vi "zoss control v1 (top level vi).vi"() -> ()   [LabVIEW 2021]
uses:
  <vilib>/Utility/error.llb/DialogType.ctl
  <vilib>/ErrorRing/Error Ring.xnode
  <vilib>/Utility/error.llb/Error Cluster From Error Code.vi
  global-variables/global variables.vi
  <extravilib>/ChannelInstances/Tag-bool.lvlib
  type-defs/maim stimulation ui states.ctl
  <vilib>/DAQmx/write.llb/DAQmx Write (Digital 1D Bool NChan 1Samp 1Line).vi
  <vilib>/DAQmx/write.llb/DAQmx Write (Digital U32 1Chan 1Samp).vi
  type-defs/stim timestamp cluster (type def).ctl
  <extravilib>/ChannelInstances/Tag-t'stim timestamp cluster (type def).ctl'.lvlib
  <extravilib>/ChannelInstances/Stream-t'sensirion_data_with_time.ctl'.lvlib
  <extravilib>/ChannelInstances/Tag-c(i32,bool).lvlib
  <vilib>/Analysis/NI_AALPro.lvlib
  <vilib>/Analysis/NI_AALBase.lvlib
  type-defs/cam_2p_status_logging_states.ctl
  <vilib>/DAQmx/read.llb/DAQmx Read (Digital 1D Bool NChan 1Samp 1Line).vi
  <vilib>/Analysis/baseanly.llb/Mean (DBL).vi
  type-defs/odor color (type def).ctl
  type-defs/stimulation configuration array (type def).ctl
  type-defs/stimulator configuration line cluster (type def).ctl
  type-defs/port-odor with color cluster (type def).ctl
  type-defs/port-odor ring (type def).ctl
  type-defs/odor and manifold config cluster (type def).ctl
  type-defs/manifold configuration cluster array (type def).ctl
  type-defs/manifold configuration cluster (type def).ctl
  type-defs/manifold selection.ctl
  type-defs/single port single odor cluster.ctl
  type-defs/port number (type def).ctl
  type-defs/odor selection (type def).ctl
  type-defs/odor description array (type def).ctl
  type-defs/odor info cluster (type def).ctl
  controls/sensirion_flow_sensor_data.ctl
  controls/sensirion_flow_sensor_data (small).ctl
panel:
  in  "DAQmx Device Name 7":tag="Dev1-USB6259"
  in  "DAQmx Device Name 6":tag="Dev1-USB6259"
  in  "DAQmx Device Name 5":tag="Dev1-USB6259"
  in  "DAQmx Device Name 4":tag="Dev1-USB6259"
  in  "DAQmx Device Name 3":tag="Dev1-USB6259"
  in  "DAQmx Device Name 2":tag="Dev1-USB6259"
  out "main progress bar":dbl(slide) scale=0.0..1.0
  out "est stim. time, s 2":dbl caption="Estimated Stimulation Duration" format="(%.0f s)"
  out "est stim. time, s":dbl caption="Estimated Stimulation Duration" format="%<%H h, %M m, %S s>t"
  out "Manual Sync":bool
  out "CAM Status":bool
  out "2P Status":bool
  out "stimulation":bool
  out "elapsed stim. time":dbl caption="Elapsed Stimulation Time" format="%<%H h, %M m, %S%1u s>t"
  out "app running":bool
  out "time":timestamp format="%<%H:%M:%S\n%x>T"
  out "experiment directory":path
  out "experiment name":string
  in  "start button":bool
  in  "quit button":bool
  in  "Tab Control":T1(tab)
  out "stim progress bar":dbl(slide)
  in  "trig on btn":bool
  in  "sol. off btn.":bool
  in  "trig off btn":bool
  in  "Trigger Selection":T2={"Trig. 0"=TRUE, "Trig. 1"=FALSE, "Trig. 2"=FALSE, "Trig. 3"=FALSE}
  out "stim duration":dbl caption="Duration" format="%<%M:%S%1u>t"
  out "Triggers":T2
  out "Stimulation Step":string
  in  "DAQmx Device Name":tag="Dev1-USB6259"
  out "Solenoid Status":T3
  out "stim status mc listbox":i32(listbox)=-1 caption="Stimulation Sequence & Status"
  out "stim loop state":T4
  in  "pre-trig pause, s (5)":dbl=5.0 caption="Pre-Trigger Pause" format="%.1f s"
  out "time left (s)":dbl caption="Time Left" format="%<%M:%S%1u>t"
  in  "post-stim pause, s (3)":dbl=3.0 caption="Post-Stimulation Pause" format="%.1f s"
  out "stim log path":path caption="Stimulation Logfile Path"
  in  "stim. run num.":i32=1 caption="Next Stimulation Run Index" format="%03d"
  out "stim. config array":T5 caption="Stimulation Sequence Configuration" {"right odor"."port-odor ring" items=["off"]; "middle odor"."port-odor ring" items=["off"=0, "fish-water (Odor: 2, Port: M.1)"=2]; "left odor"."port-odor ring" items=["off"]}
  in  "config stim button":bool
  out "odor & manifold config cluster":T10
  in  "config odor-manifold button":bool
  in  "dish volume live?":bool=TRUE caption="Live Volume"
  in  "dish volume input":dbl[unit] format="%0.2f"
  out "dish vol.":dbl[unit](slide) caption="Dish Volume (mL)"
  out "sensor uptime":dbl[unit] caption="Sensor Log Up-Time" format="%<%H h, %M m, %S%1u s>t"
  out "Sensor Status":errorcluster
  in  "sensor monitor stop-start":bool
  out "wash-vac delta":dbl[unit](slide) caption="Dish Net Flow Rate"
  out "10 sensor data clustor":T20={"sensor 0"={"flow rate \n"=0.0, "flow val. status"=FALSE, "temperature"=273.15, "temp. val status"=FALSE, "air in line?"=FALSE, "high flow?"=FALSE, "flag. val status"=FALSE}, "sensor 1"={"flow rate \n"=0.0, "flow val. status"=FALSE, "temperature"=273.15, "temp. val status"=FALSE, "air in line?"=FALSE, "high flow?"=FALSE, "flag. val status"=FALSE}, "sensor 2"={"flow rate \n"=0.0, "flow val. status"=FALSE, "temperature"=273.15, "temp. val status"=FALSE, "air in line?"=FALSE, "high flow?"=FALSE, "flag. val status"=FALSE}, "sensor 3"={"flow rate \n"=0.0, "flow val. status"=FALSE, "temperature"=273.15, "temp. val status"=FALSE, "air in line?"=FALSE, "high flow?"=FALSE, "flag. val status"=FALSE}, "sensor 4"={"flow rate \n"=0.0, "flow val. status"=FALSE, "temperature"=273.15, "temp. val status"=FALSE, "air in line?"=FALSE, "high flow?"=FALSE, "flag. val status"=FALSE}, "sensor 5"={"flow rate \n"=0.0, "flow val. status"=FALSE, "temperature"=273.15, "temp. val status"=FALSE, "air in line?"=FALSE, "high flow?"=FALSE, "flag. val status"=FALSE}, "sensor 6"={"flow rate \n"=0.0, "flow val. status"=FALSE, "temperature"=273.15, "temp. val status"=FALSE, "air in line?"=FALSE, "high flow?"=FALSE, "flag. val status"=FALSE}, "sensor 7"={"flow rate \n"=0.0, "flow val. status"=FALSE, "temperature"=273.15, "temp. val status"=FALSE, "air in line?"=FALSE, "high flow?"=FALSE, "flag. val status"=FALSE}, "sensor 8"={"flow rate \n"=0.0, "flow val. status"=FALSE, "temperature"=273.15, "temp. val status"=FALSE, "air in line?"=FALSE, "high flow?"=FALSE, "flag. val status"=FALSE}, "sensor 9"={"flow rate \n"=0.0, "flow val. status"=FALSE, "temperature"=273.15, "temp. val status"=FALSE, "air in line?"=FALSE, "high flow?"=FALSE, "flag. val status"=FALSE}} {"sensor 9"."temperature" scale=293.15..303.15 scale format="%#_3g"; "sensor 8"."temperature" scale=293.15..303.15 scale format="%#_3g"; "sensor 7"."temperature" scale=293.15..303.15 scale format="%#_3g"; "sensor 6"."temperature" scale=293.15..303.15 scale format="%#_3g"; "sensor 5"."temperature" scale=293.15..303.15 scale format="%#_3g"; "sensor 4"."temperature" scale=293.15..303.15 scale format="%#_3g"; "sensor 3"."temperature" scale=293.15..303.15 scale format="%#_3g"; "sensor 2"."temperature" scale=293.15..303.15 scale format="%#_3g"; "sensor 1"."temperature" scale=293.15..303.15 scale format="%#_3g"; "sensor 0"."temperature" scale=293.15..303.15 scale format="%#_3g"}
  out "sensor 10 (wash)":T21={"flow rate \n"=0.0, "flow val. status"=FALSE, "temperature"=273.15, "temp. val status"=FALSE, "air in line?"=FALSE, "high flow?"=FALSE, "flag. val status"=FALSE} caption="Wash Line Data (11)" {"temperature" scale=293.15..303.15 scale format="%#_3g"}
  out "sensor 11 (vacuum)":T21={"flow rate \n"=0.0, "flow val. status"=FALSE, "temperature"=273.15, "temp. val status"=FALSE, "air in line?"=FALSE, "high flow?"=FALSE, "flag. val status"=FALSE} caption="Vacuum Line Data (12)" {"temperature" scale=293.15..303.15 scale format="%#_3g"}
  in  "Arduino COM Port":refnum<visa-resource-name>="COM3"
  in  "simulate?":bool caption="SIM"
  out "flow sense path":path caption="Flow Sensor Logfile Path"
  out "smp rate":dbl[unit] caption="Average Sampling Rate"
  in  "mov. mean size (3)":u32=3 caption="Moving\nAverage\nWidth"
  out "wash-vac flow rate \nxy graph":cluster{"X":dbl[], "Y":dbl[]}[](graph)
  # "Time"
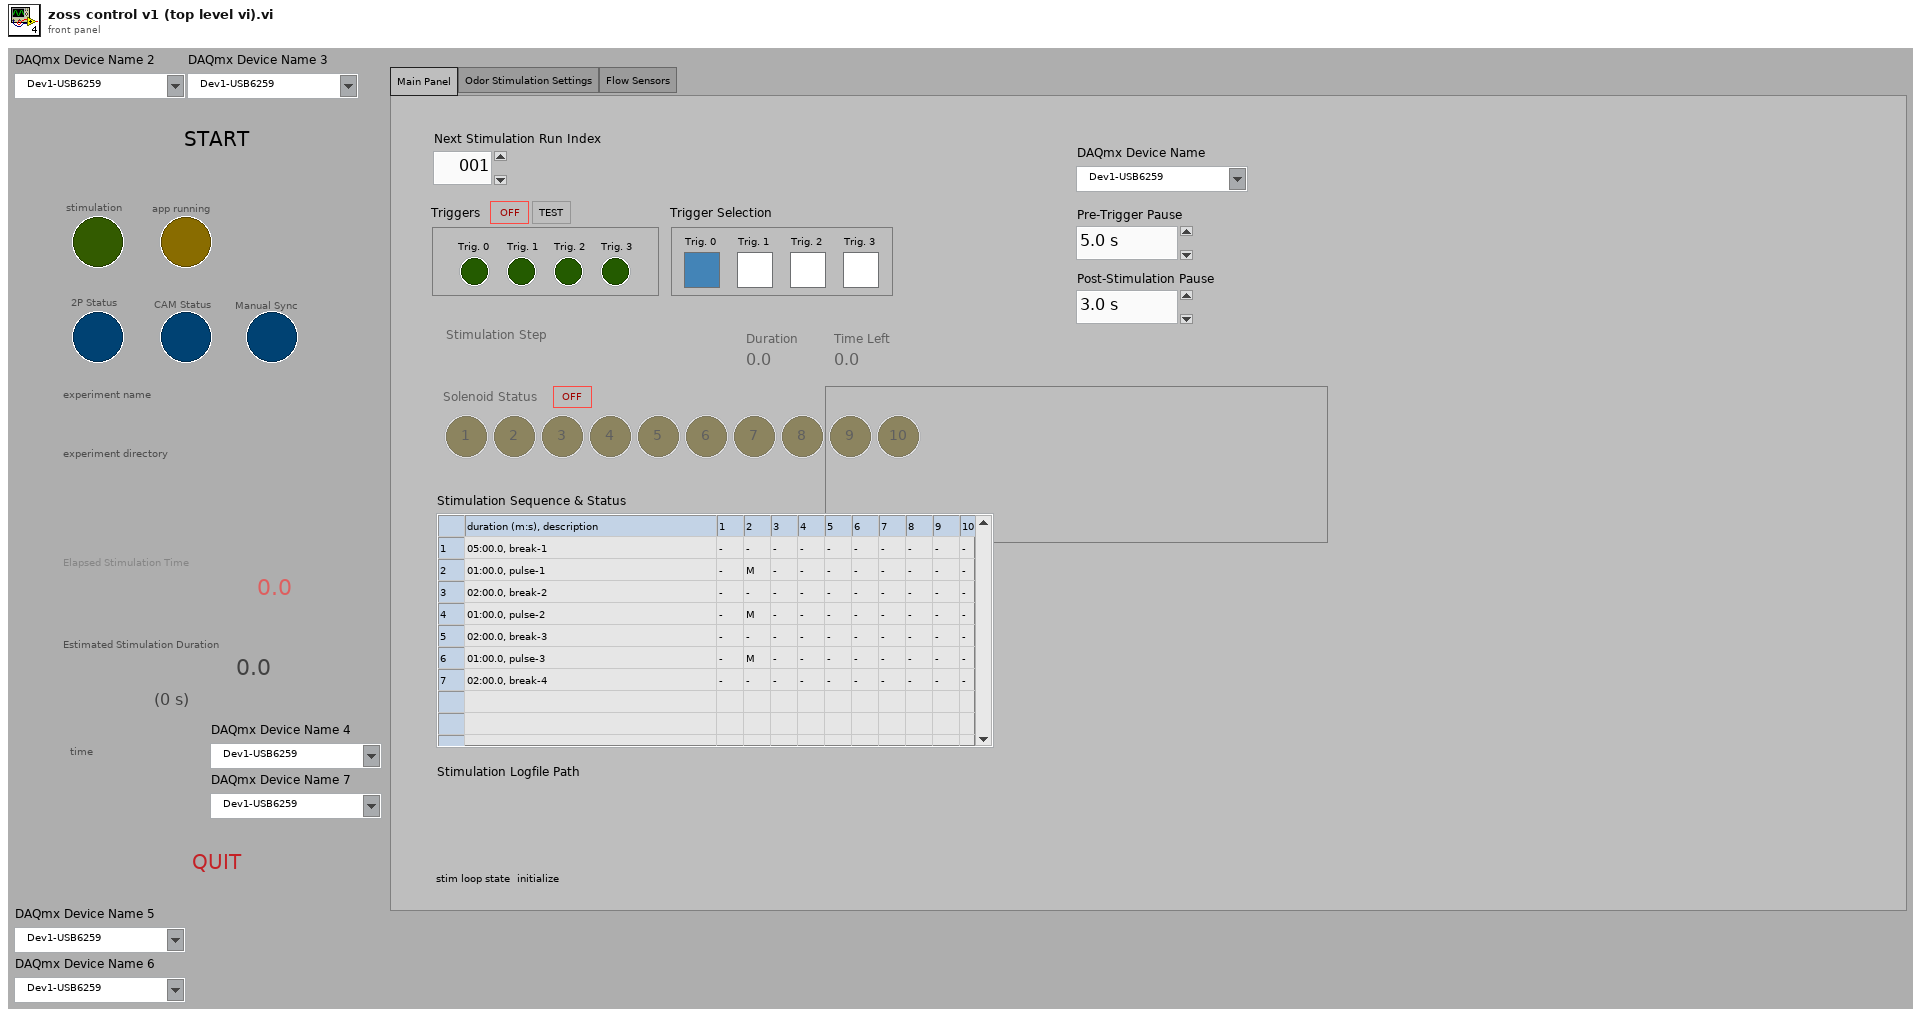
[diagram p1: front panel]
types:
  T1 = enum32{"Main Panel", "Odor Stimulation Settings", "Flow Sensors"}
  T2 = cluster{"Trig. 0":bool, "Trig. 1":bool, "Trig. 2":bool, "Trig. 3":bool}
  T3 = cluster{"Boolean":bool, "Boolean 2":bool, "Boolean 3":bool, "Boolean 4":bool, "Boolean 5":bool, "Boolean 6":bool, "Boolean 7":bool, "Boolean 8":bool, "Boolean 9":bool, "Boolean 10":bool}
  T4 = typedef "maim stimulation ui states.ctl" = enum16{"initialize", "idle", "update listbox", "wait for event", "countdown", "trigger hardware", "perform stimulation", "end stimulation", "update nidaq task", "exit"}
  T5 = typedef "stimulation configuration array (type def).ctl" = T6[]
  T6 = typedef "stimulator configuration line cluster (type def).ctl" = cluster{"description":string, "duration, s":dbl, "left odor":T7, "middle odor":T7, "right odor":T7, "selected?":bool}
  T7 = typedef "port-odor with color cluster (type def).ctl" = cluster{"port-odor ring":T8, "odor color":T9}
  T8 = typedef "port-odor ring (type def).ctl" = u16
  T9 = typedef "odor color (type def).ctl" = u16
  T10 = typedef "odor and manifold config cluster (type def).ctl" = cluster{"manifold config":T11, "odor config":T17}
  T11 = typedef "manifold configuration cluster array (type def).ctl" = T12[]
  T12 = typedef "manifold configuration cluster (type def).ctl" = cluster{"position:":T13, "port connections:":T14[]}
  T13 = typedef "manifold selection.ctl" = enum16{"left", "middle", "right"}
  T14 = typedef "single port single odor cluster.ctl" = cluster{"port number":T15, "connected odor":T16, "error":bool, "odor color":T9}
  T15 = typedef "port number (type def).ctl" = enum16{"port 1", "port 2", "port 3", "port 4", "port 5", "port 6", "port 7", "port 8"}
  T16 = typedef "odor selection (type def).ctl" = enum16{"[none]", "odor 1", "odor 2", "odor 3", "odor 4", "odor 5", "odor 6", "odor 7", "odor 8", "odor 9", "odor 10"}
  T17 = typedef "odor description array (type def).ctl" = T18[]
  T18 = typedef "odor info cluster (type def).ctl" = cluster{"odor channel":T16, "odor description":string, "odor color":T9, "odor channel active":bool}
  T19 = typedef "sensirion_flow_sensor_data (small).ctl" = cluster{"flow rate \n":dbl[unit], "flow val. status":bool, "temperature":dbl[unit], "temp. val status":bool, "air in line?":bool, "high flow?":bool, "flag. val status":bool}
  T20 = cluster{"sensor 0":T19, "sensor 1":T19, "sensor 2":T19, "sensor 3":T19, "sensor 4":T19, "sensor 5":T19, "sensor 6":T19, "sensor 7":T19, "sensor 8":T19, "sensor 9":T19}
  T21 = typedef "sensirion_flow_sensor_data.ctl" = cluster{"flow rate \n":dbl[unit], "flow val. status":bool, "temperature":dbl[unit], "temp. val status":bool, "air in line?":bool, "high flow?":bool, "flag. val status":bool}
  T22 = typedef "cam_2p_status_logging_states.ctl" = enum16{"initialize", "idle", "wait for stim begin", "prepare for log", "log", "end log", "exit"}
  T23 = typedef "DialogType.ctl" = u16
  T24 = enum8{"Enabled", "Disabled", "Disabled and Grayed Out"}
  T25 = typedef "Tag-bool.lvlib/))Channel.ctl" = refnum<queue>
  T26 = typedef "LVDateTimeRec.ctl" = cluster{"fractional second":dbl, "second":i32, "minute":i32, "hour":i32, "day of month":i32, "month":i32, "year":i32, "day of week":i32, "day of year":i32, "DST":i32}
  T27 = cluster{"[0]":bool, "[1]":bool, "[2]":bool, "[3]":bool}
  T28 = cluster{"[0]":bool, "[1]":bool, "[2]":bool, "[3]":bool, "[4]":bool, "[5]":bool, "[6]":bool, "[7]":bool, "[8]":bool, "[9]":bool}
  T29 = typedef "Tag-c(i32,bool).lvlib/))Channel.ctl" = refnum<queue>
  T30 = enum16{"open", "replace", "create", "open or create", "replace or create", "replace or create with confirmation"}
  T31 = typedef "Stream-t'sensirion_data_with_time.ctl'.lvlib/)Channel.ctl" = refnum<queue>
  T32 = typedef "sensirion_data_with_time.ctl" = cluster{"sensor data array":T21[], "relative timestamp":dbl, "error":errorcluster}
  T33 = cluster{"[0]":T21, "[1]":T21, "[2]":T21, "[3]":T21, "[4]":T21, "[5]":T21, "[6]":T21, "[7]":T21, "[8]":T21, "[9]":T21}
  T34 = typedef "stim timestamp cluster (type def).ctl" = cluster{"valid?":bool, "rel. time, s":dbl, "index":i32}
  T35 = cluster{"Trigger Selection[0]":bool, "Trigger Selection[1]":bool, "Trigger Selection[2]":bool, "Trigger Selection[3]":bool}
  T36 = typedef "Tag-t'stim timestamp cluster (type def).ctl'.lvlib/))Channel.ctl" = refnum<queue>
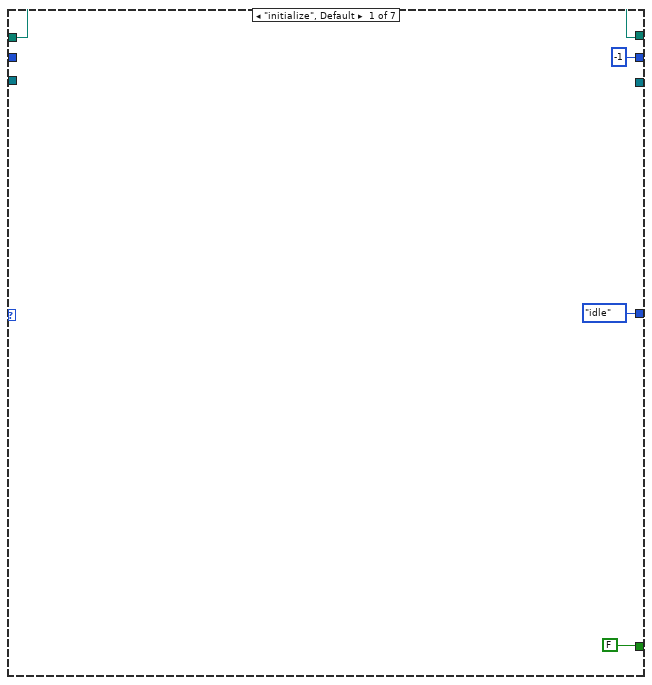
[diagram p2: hidden frame]
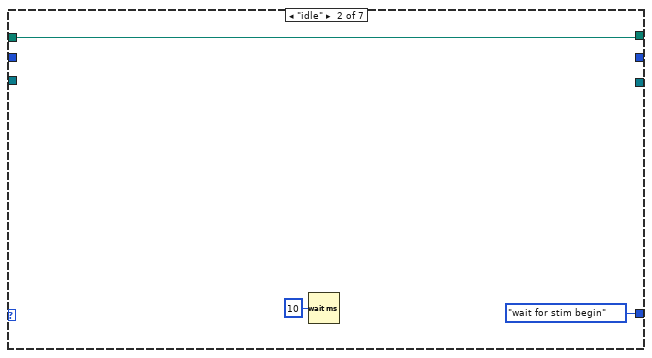
[diagram p3: hidden frame]
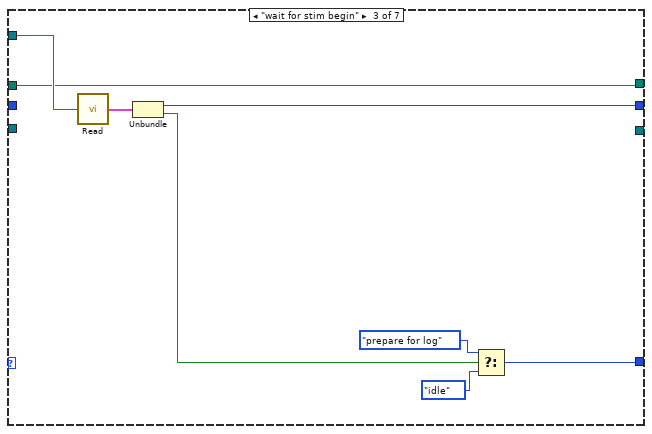
[diagram p4: hidden frame]
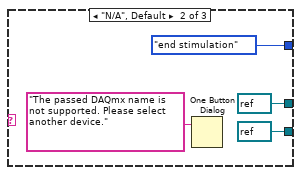
[diagram p5: hidden frame]
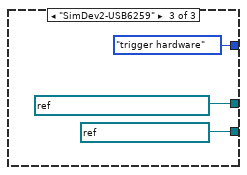
[diagram p6: hidden frame]
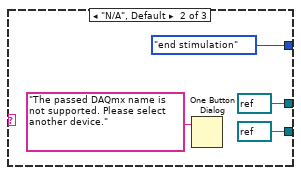
[diagram p7: hidden frame]
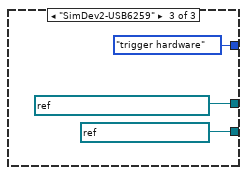
[diagram p8: hidden frame]
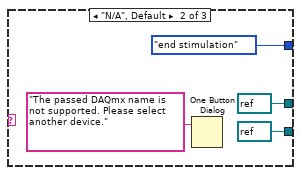
[diagram p9: hidden frame]
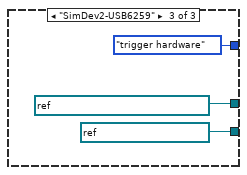
[diagram p10: hidden frame]
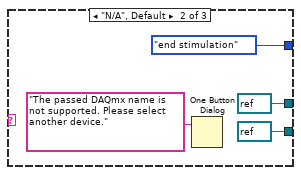
[diagram p11: hidden frame]
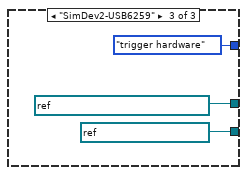
[diagram p12: hidden frame]
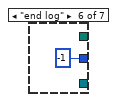
[diagram p14: hidden frame]
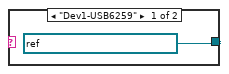
[diagram p16: hidden frame]
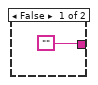
[diagram p17: hidden frame]
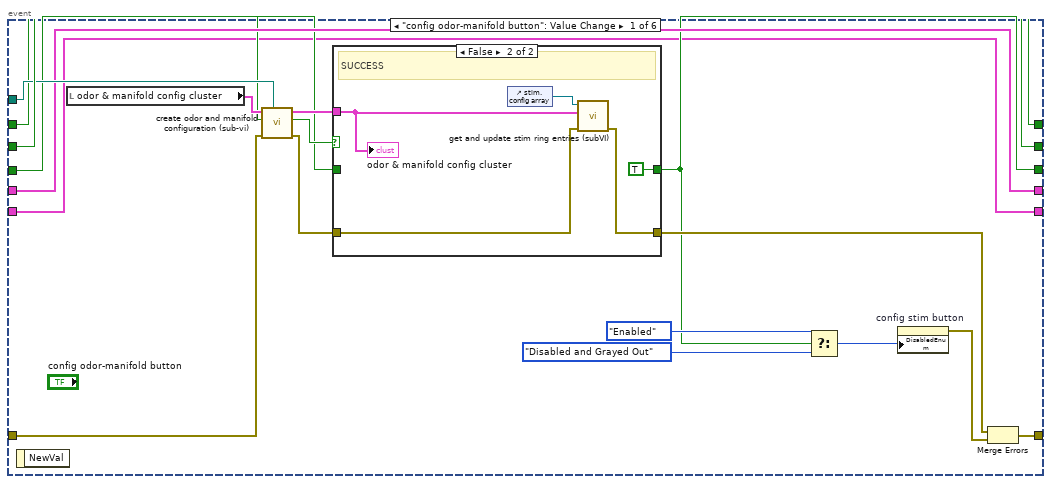
[diagram p19: hidden frame]
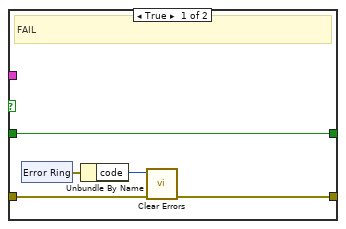
[diagram p20: hidden frame]
diagram:
  w31 = T23 2 items=["no dialog", "OK message", "continue or stop message", "OK message + warnings", "continue/stop + warnings"] ("type of dialog (OK msg:1)")
  n1 = flat-sequence "Initialization Tasks" {
    tunnel: [w60] -> w14
    frame #0 {
      n2 = control-ref of="This VI"() -> (w33:refnum<vi>)
      n3 = invoke on="Invoke Node" class="VI" method="Default Vals.Reinit All"(reference=w33) -> ()  [unwired: 2 in, 3 out]
    }
    frame #1 {
      w34 = T24."Disabled" ("Disabled")
      w35 = FALSE ("Visible")
      w39 = T24."Enabled" ("Disabled")
      w36 = T24."Enabled" ("Disabled")
      w63 = T24."Disabled" ("Disabled")
      n4 = property on="DAQmx Device Name" class="DAQmxName"() -> ("Value"=w40:string)  [unwired: 2 in, 2 out]
      n5 = property on="stim. run num." class="DigNum (strict)"("DisabledEnum"=T24."Enabled" ("Disabled"), "Caption.Text"="Next Stimulation Run Index") -> ()  [unwired: 2 in, 2 out]
      n6 = property on="trig off btn" class="Bool (strict)"("Val(Sgnl)"=TRUE) -> ()  [unwired: 2 in, 2 out]
      n7 = property on="sol. off btn." class="Bool (strict)"("Val(Sgnl)"=TRUE) -> ()  [unwired: 2 in, 2 out]
      n8 = property on="DAQmx Device Name" class="DAQmxName"("Val(Sgnl)"=w40) -> ()  [unwired: 2 in, 2 out]
      n9 = property on="trig off btn" class="Bool (strict)"("DisabledEnum"=w39) -> ()  [unwired: 2 in, 2 out]
      n10 = property on="trig on btn" class="Bool (strict)"("DisabledEnum"=w39) -> ()  [unwired: 2 in, 2 out]
      n11 = property on="sol. off btn." class="Bool (strict)"("DisabledEnum"=w39) -> ()  [unwired: 2 in, 2 out]
      n12 = property on="DAQmx Device Name" class="DAQmxName"("DisabledEnum"=w36) -> ()  [unwired: 2 in, 2 out]
      n13 = property on="Trigger Selection" class="Clust (strict)"("DisabledEnum"=w36) -> ()  [unwired: 2 in, 2 out]
      n14 = property on="main progress bar" class="Slide (strict)"("Visible"=w35, "DisabledEnum"=w34) -> ()  [unwired: 2 in, 2 out]
      n15 = property on="stim progress bar" class="Slide (strict)"("Visible"=w35, "DisabledEnum"=w34) -> ()  [unwired: 2 in, 2 out]
      n16 = property on="Stimulation Step" class="Str"("DisabledEnum"=T24."Disabled and Grayed Out" ("Disabled")) -> ()  [unwired: 2 in, 2 out]
      n17 = local read "dish volume live?"() -> (w59:bool)
      n18 = control-ref of="stim status mc listbox"() -> (w53:refnum<vi>)
      n19 = Not(x=w59) -> (.not. x?=w57:bool)
      n20 = call "bool to disabled state (sub-vi).vi"("error?"=w57) -> ("disabled"=w58:T24)
      n21 = call "bool to disabled state (sub-vi).vi"("error?"=w59) -> ("disabled"=w56:T24)
      n22 = local write "stim duration"(nan ("stim duration")) -> ()
      n23 = local write "time left (s)"(nan ("time left (s)")) -> ()
      n24 = property on="stim. config array" class="Arr (strict)"("Index Values"=u32[] [0], "DisabledEnum"=w63) -> (error out=w67:errorcluster)  [unwired: 2 in, 1 out]
      n25 = property on="time left (s)" class="DigNum (strict)"("DisabledEnum"=T24."Disabled and Grayed Out" ("Disabled")) -> ()  [unwired: 2 in, 2 out]
      n26 = property on="stim duration" class="DigNum (strict)"("DisabledEnum"=T24."Disabled and Grayed Out" ("Disabled")) -> ()  [unwired: 2 in, 2 out]
      n27 = property on="dish volume input" class="DigNum (strict)"("DisabledEnum"=w56) -> ()  [unwired: 2 in, 2 out]
      n28 = property on="dish vol." class="Slide (strict)"("DisabledEnum"=w58) -> ()  [unwired: 2 in, 2 out]
      n29 = property on="config odor-manifold button" class="Bool"("DisabledEnum"=T24."Enabled" ("Disabled")) -> (error out=w69:errorcluster)  [unwired: 2 in, 1 out]
      n30 = property on="Solenoid Status" class="Clust (strict)"("DisabledEnum"=T24."Disabled and Grayed Out" ("Disabled")) -> ()  [unwired: 2 in, 2 out]
      n31 = property on="start button" class="Bool"("DisabledEnum"=T24."Disabled and Grayed Out" ("Disabled")) -> (error out=w68:errorcluster)  [unwired: 2 in, 1 out]
      n32 = property on="elapsed stim. time" class="DigNum (strict)"("DisabledEnum"=T24."Disabled and Grayed Out" ("Disabled"), "Blinking"=FALSE) -> ()  [unwired: 2 in, 2 out]
      n33 = property on="odor & manifold config cluster" class="Clust (strict)"("DisabledEnum"=w63) -> ()  [unwired: 2 in, 2 out]
      n34 = property on="config stim button" class="Bool"("DisabledEnum"=T24."Disabled and Grayed Out" ("Disabled")) -> (error out=w66:errorcluster)  [unwired: 2 in, 1 out]
      n35 = call "init mc listbox stimulation status (subVI).vi"("mc listbox refnum"=w53, "font size (16)"=u32 18, "num visible rows (8)"=u32 10, "cell width (35)"=u32 25, "description cell width (150)"=u32 250) -> ()  [unwired: 9 in, 2 out]
      n36 = Merge Errors(w69, w68, w67, w66) -> (w60:errorcluster)
    }
  }
  n37 = call "Untitled 1.vi"("error in (no error)"=w14) -> ("Append datetime stamp?"=w22:bool, "Experiment Name"=w28:string, "error out"=w23:errorcluster)  [unwired: 15 in, 1 out]
  n38 = Empty String/Path?(string/path=w28) -> (empty?=w29:bool)
  n39 = case shown="True" w22 {
    tunnel: ["" w72] -> w20
    frame False {
    }
    frame True {
      n40 = Format Date/Time String(time format string (%c)="_%Y%m%d-%H%M") -> (date/time string=w72:string)  [unwired: 2 in]
    }
  }
  n41 = case shown="True" w29 {
    tunnel: w28 -> [w73 _]
    tunnel: [w73 "no-nb-ref-(untitled)"] -> w25
    frame False {
    }
    frame True {
    }
  }
  "experiment name" <- w25
  n42 = global read "global variables.vi" "default data directory"() -> (w24:path)
  n43 = Format Into String(format string="_zoss-system-data%s" ("time format string (%c)"), w20) -> (resulting string=w19:string)  [unwired: 2 in, 1 out]
  n44 = Concatenate Strings(w25, w19) -> (w27:string)
  n45 = String To Path(string=w27) -> (path=w26:path)
  n46 = Build Path(base path=w24, name or relative path=w26) -> (appended path=w18:path)
  n47 = call "handle input dir with subdir (subVI).vi"("error in (no error)"=w23, "starting directory (none)"=w18) -> ("error out"=w17:errorcluster, "dirctory path"=w3:path)  [unwired: 8 in]
  "experiment directory" <- w3
  n48 = flat-sequence {
    tunnel: [TRUE] -> w8
    frame #0 {
      n49 = event "Stop Execution" shown="[0] \"quit button\": Value Change" {
        selector: _ -> [_]
        dyn-events: _ -> [_]
        timeout: _ -> [_]
        event "quit button": Value Change {
          n50 = event-data() -> ()  [unwired: 1 in, 1 out]
        }
      }
    }
    frame #1 {
      n51 = call <vilib>:"Set Busy.vi"() -> ()  [unwired: 10 in, 2 out]
      n52 = property on="trig off btn" class="Bool (strict)"("Val(Sgnl)"=TRUE) -> ()  [unwired: 2 in, 2 out]
      n53 = property on="sol. off btn." class="Bool (strict)"("Val(Sgnl)"=TRUE) -> ()  [unwired: 2 in, 2 out]
      n54 = Wait (ms)(milliseconds to wait=u32 50) -> ()  [unwired: 1 out]
    }
    frame #2 {
      n55 = Wait (ms)(milliseconds to wait=u32 50) -> ()  [unwired: 1 out]
    }
    frame #3 {
      n56 = call <vilib>:"Unset Busy.vi"() -> ()  [unwired: 11 in, 1 out]
    }
    frame #4 {
      n57 = Stop() -> ()  [unwired: 1 in]
    }
  }
  n58 = call <vilib>:"Simple Error Handler.vi"("type of dialog (OK msg:1)"=w31, "error in (no error)"=w17) -> ()  [unwired: 3 in, 5 out]
  n59 = call <extravilib>:"Write.vi"("element"=w8) -> ("channel"=w1:T25)  [unwired: 1 out]
  n60 = while {
    tunnel: w1 -> [w81]
    stop <- w80 stop-if-true
    # "Time and Running Display"
    n61 = local read "DAQmx Device Name"() -> (w87:tag)
    n62 = call <extravilib>:"Read.vi"("channel"=w81) -> ("element"=w80:bool)  [unwired: 1 in, 1 out]
    n63 = case shown="\"SimDev2-USB6259\", Default" w87 {
      tunnel: [refnum<k21> "Dev1-6259_DigIn_P1_L4-7" refnum<k21> "Sim6259_DigIn_P1_L4-7"] -> w86
      frame "Dev1-USB6259" {
      }
      frame "SimDev2-USB6259", Default {
      }
    }
    n64 = Get Date/Time In Seconds() -> (seconds since 1Jan1904=w92:timestamp)
    "time" <- w92
    n65 = Wait (ms)(milliseconds to wait=u32 100) -> ()  [unwired: 1 out]
    n66 = Seconds To Date/Time(time stamp (now)=w92) -> (date time rec=w91:T26)  [unwired: 1 in]
    n67 = Unbundle By Name(w91) -> ("fractional second"=w88:dbl)
    n68 = Less?(x=w88, y=0.5) -> (x < y?=→"app running":bool)
    n69 = call-poly <vilib>:"DAQmx Read.vi"("task/channels in"=w86) -> ("data"=w85:bool[])  [unwired: 12 in, 2 out]
    n70 = Index Array(array=w85) -> (element #1=→"2P Status":bool, element #2=→"CAM Status":bool, element #3=→"Manual Sync":bool)  [unwired: 3 in]
  }
  n71 = call <extravilib>:"Write.vi"("element"=FALSE, "channel"=w1) -> ()  [unwired: 1 out]
  n72 = while {
    shift-right: [w106] -> _
    shift-left: FALSE -> [w119]
    shift-right: [w110] -> _
    shift-left: w17 -> [w117]
    shift-right: [w107] -> _
    shift-left: FALSE -> [w116]
    tunnel: w3 -> [w115]
    shift-right: [w114] -> _
    shift-left: _ -> [w113]
    shift-right: [w108] -> _
    shift-left: FALSE -> [w109]
    tunnel: w1 -> [w102]
    shift-right: [w97] -> _
    shift-left: _ -> [w96]
    stop <- w101 stop-if-true
    w118 = T23 2 items=["no dialog", "OK message", "continue or stop message", "OK message + warnings", "continue/stop + warnings"] ("type of dialog (OK msg:1)")
    # "Odor, Manifold, and Stimulation Configuration Interaction"
    n73 = call <extravilib>:"Read.vi"("channel"=w102) -> ("element"=w101:bool)  [unwired: 1 in, 1 out]
    n74 = event shown="[4] \"trig on btn\": Value Change" {
      selector: _ -> [_ _ _ _ _ _]
      dyn-events: _ -> [_ _ _ _ _ _]
      timeout: _ -> [_ _ _ _ _ _]
      tunnel: w119 -> [w123 w159 w199 w217 w228 w251]
      tunnel: [w122 w159 w199 w217 w228 w251] -> w106
      tunnel: [w130 w160 w198 w216 w227 w256] -> w111
      tunnel: w117 -> [w131 w164 w198 w216 w227 w256]
      tunnel: w116 -> [w128 w156 w197 w215 w226 w252]
      tunnel: [w128 w155 w197 w215 w226 w252] -> w107
      tunnel: w115 -> [w125 w153 _ _ _ _]
      tunnel: [w124 w157 w196 w214 w225 w250] -> w114
      tunnel: w113 -> [w124 w158 w196 w214 w225 w250]
      tunnel: [w121 w154 w195 w213 w224 w254] -> w108
      tunnel: w109 -> [w121 w154 w195 w213 w224 _]
      tunnel: [w120 w152 w187 w203 w221 w238] -> w97
      tunnel: w96 -> [w120 w152 _ w203 w222 w238]
      event "config odor-manifold button": Value Change {
        n75 = event-data() -> ()  [unwired: 1 in, 1 out]
        n76 = local read "odor & manifold config cluster"() -> (w135:T10)
        n77 = call "create odor and manifold configuration (sub-vi).vi"("default directory (none)"=w125, "error in (no error)"=w131, "use initial config? (F)"=w123, "initial odor and manifold config (none)"=w135) -> ("error out"=w129:errorcluster, "operation failed?"=w136:bool, "odor and manifold config out"=w137:T10)  [unwired: 5 in]
        n78 = case shown="False" w136 {
          tunnel: w137 -> [_ w150]
          tunnel: w123 -> [w142 _]
          tunnel: [w142 TRUE] -> w122
          tunnel: w129 -> [w139 w148]
          tunnel: [w138 w147] -> w126
          frame True {
            # "FAIL"
            n79 = xnode "Error Ring"() -> ("error out"=w141:errorcluster)
            n80 = Unbundle By Name(w141) -> ("code"=w140:i32)
            n81 = call <vilib>:"Clear Errors.vi"("error in (no error)"=w139, "specific error code to clear (0: all)"=w140) -> ("error out"=w138:errorcluster)  [unwired: 4 in, 1 out]
          }
          frame False {
            # "SUCCESS"
            n82 = control-ref of="stim. config array"() -> (w149:refnum<vi>)
            n83 = call "get and update stim ring entries (subVI).vi"("error in (no error)"=w148, "odor-manifold config"=w150, "stim config array refnum"=w149) -> ("error out"=w147:errorcluster)  [unwired: 7 in, 1 out]
            "odor & manifold config cluster" <- w150
          }
        }
        n84 = Select(t=T24."Enabled" ("Disabled"), s=w122, f=T24."Disabled and Grayed Out" ("Disabled")) -> (s? t:f=w133:T24)
        n85 = property on="config stim button" class="Bool"("DisabledEnum"=w133) -> (error out=w127:errorcluster)  [unwired: 2 in, 1 out]
        n86 = Merge Errors(w126, w127) -> (w130:errorcluster)
      }
      event "config stim button": Value Change {
        n87 = event-data() -> ()  [unwired: 1 in, 2 out]
        n88 = local read "odor & manifold config cluster"() -> (w166:T10)
        n89 = local read "stim. config array"() -> (w165:T5)
        n90 = call "configure stimulation dialog (subVI).vi"("default directory (none)"=w153, "error in (no error)"=w164, "use initial config? (F)"=w156, "odor and manifold config"=w166, "initial stim. config [] (empty array)"=w165) -> ("error out"=w161:errorcluster, "operation failed?"=w162:bool, "stim. config [] out"=w163:T5)  [unwired: 4 in]
        n91 = case shown="False" w162 {
          tunnel: w163 -> [w170 _]
          tunnel: w161 -> [w175 w180]
          tunnel: [w175 w179] -> w160
          tunnel: [TRUE w177] -> w155
          tunnel: [w170 w178] -> w157
          tunnel: w158 -> [_ w178]
          tunnel: w156 -> [_ w177]
          frame False {
            # "SUCCESS"
            n92 = control-ref of="stim status mc listbox"() -> (w171:refnum<vi>)
            n93 = call "stim config array to description array (subVI).vi"("add duration? (F)"=TRUE, "stim. config array"=w170) -> ("description []"=w174:string[])  [unwired: 9 in]
            n94 = call "stim config array to bool odor matrix (subVI).vi"("stim. config []"=w170) -> ("string stim. matrix"=w172:string[][], "bool stim. matrix"=w173:bool[][], "duration []"=w168:dbl[])  [unwired: 8 in]
            n95 = call "update mc lsitbox from stim config (subVI).vi"("description []"=w174, "string stim. matrix"=w172, "bool stim. matrix"=w173, "mc listbox refnum"=w171) -> ()  [unwired: 6 in, 2 out]
            n96 = Add Array Elements(numeric array=w168) -> (sum=→"est stim. time, s" →"est stim. time, s 2":dbl)
            "stim. config array" <- w170
          }
          frame True {
            # "FAIL"
            n97 = xnode "Error Ring"() -> ("error out"=w182:errorcluster)
            n98 = Unbundle By Name(w182) -> ("code"=w181:i32)
            n99 = call <vilib>:"Clear Errors.vi"("error in (no error)"=w180, "specific error code to clear (0: all)"=w181) -> ("error out"=w179:errorcluster)  [unwired: 4 in, 1 out]
          }
        }
      }
      event "trig off btn": Value Change {
        n100 = event-data() -> ()  [unwired: 1 in, 5 out]
        n101 = case shown="True" "trig off btn" {
          frame False {
          }
          frame True {
            n102 = local write "trig off btn"(FALSE ("trig off btn")) -> ()
          }
        }
        n103 = local read "DAQmx Device Name"() -> (w193:tag)
        n104 = case shown="\"SimDev2-USB6259\", Default" w193 {
          tunnel: [refnum<k21> "Dev1-6259_TriggerOut_P1_L0-3" refnum<k21> "Sim6259_TriggerOut_P1_L0-3"] -> w192
          frame "Dev1-USB6259" {
          }
          frame "SimDev2-USB6259", Default {
          }
        }
        n105 = Initialize Array(FALSE, 4 ("dimension size")) -> (w188:bool[])
        n106 = Array To Cluster(array=w188) -> (cluster=w187:T27)
        n107 = call-poly <vilib>:"DAQmx Write.vi"("task/channels in"=w192, "auto start"=TRUE, "data"=w188) -> ()  [unwired: 10 in, 3 out]
        n108 = local write "Triggers"(w187) -> ()
      }
      event "sol. off btn.": Value Change {
        w205 = u32 0 ("data")
        n109 = event-data() -> ()  [unwired: 1 in, 5 out]
        n110 = case shown="True" "sol. off btn." {
          frame False {
          }
          frame True {
            n111 = local write "sol. off btn."(FALSE ("sol. off btn.")) -> ()
          }
        }
        n112 = local read "DAQmx Device Name"() -> (w211:tag)
        n113 = case shown="\"Dev1-USB6259\"" w211 {
          tunnel: [refnum<k21> "Dev1-6259_DigOut_P0" refnum<k21> "Sim6259_DigOut_P0"] -> w210
          frame "Dev1-USB6259" {
          }
          frame "SimDev2-USB6259", Default {
          }
        }
        n114 = Number To Boolean Array(number=w205) -> (Boolean array=w208:bool[])
        n115 = call-poly <vilib>:"DAQmx Write.vi"("task/channels in"=w210, "auto start"=TRUE, "data"=w205) -> ()  [unwired: 10 in, 3 out]
        n116 = Array Subset(array=w208, length=10) -> (w207:bool[])  [unwired: 1 in]
        n117 = Array To Cluster(array=w207) -> (cluster=w204:T28)
        n118 = local write "Solenoid Status"(w204) -> ()
      }
      event "trig on btn": Value Change {
        n119 = event-data() -> ()  [unwired: 1 in, 5 out]
        n120 = case shown="False" "trig on btn" {
          tunnel: [w230 w231] -> w221
          tunnel: w222 -> [w230 _]
          frame False {
            n121 = property on="trig off btn" class="Bool (strict)"("Val(Sgnl)"=TRUE) -> ()  [unwired: 2 in, 2 out]
          }
          frame True {
            n122 = local read "DAQmx Device Name"() -> (w235:tag)
            n123 = case shown="\"SimDev2-USB6259\", Default" w235 {
              tunnel: [refnum<k21> "Dev1-6259_TriggerOut_P1_L0-3" refnum<k21> "Sim6259_TriggerOut_P1_L0-3"] -> w234
              frame "Dev1-USB6259" {
              }
              frame "SimDev2-USB6259", Default {
              }
            }
            n124 = local read "Trigger Selection"() -> (w231:T2)
            n125 = Cluster To Array(cluster=w231) -> (array=w232:bool[])
            n126 = local write "Triggers"(w231) -> ()
            n127 = call-poly <vilib>:"DAQmx Write.vi"("task/channels in"=w234, "auto start"=TRUE, "data"=w232) -> ()  [unwired: 10 in, 3 out]
          }
        }
      }
      event "DAQmx Device Name": Value Change {
        n128 = event-data() -> ("OldVal"=w253:tag, "NewVal"=w245:tag)  [unwired: 1 in]
        n129 = global read "global variables.vi" "valid DAQmx device []"() -> (w249:string[])
        n130 = node("") -> (w243:set{string})
        n131 = for {
          tunnel: w249 -> [w259] mode=indexing
          shift-right: [w257] -> w248
          shift-left: w243 -> [w258]
          n132 = Insert Into Set(10:w259, 11:w258) -> (3:w257:set{string})  [unwired: 1 out]
        }
        n133 = Type Cast(type="", x=w245) -> (*(type *) &x=w242:string)
        n134 = Element of Set?(10:w242, 11:w248) -> (3:w246:bool)
        n135 = case shown="False" w246 {
          tunnel: w253 -> [_ w263]
          tunnel: w245 -> [w262 _]
          tunnel: w242 -> [_ w264]
          tunnel: [w262 w263] -> w240
          frame True {
            n136 = property on="trig off btn" class="Bool (strict)"("Val(Sgnl)"=TRUE) -> ()  [unwired: 2 in, 2 out]
            n137 = property on="sol. off btn." class="Bool (strict)"("Val(Sgnl)"=TRUE) -> ()  [unwired: 2 in, 2 out]
          }
          frame False {
            n138 = local write "DAQmx Device Name"(w263) -> ()
            n139 = Format Into String(format string="The passed device, \"%s\", is not supported. Please select another device." ("message"), w264) -> (resulting string=w266:string)  [unwired: 2 in, 1 out]
            n140 = One Button Dialog(message=w266) -> ()  [unwired: 1 in, 1 out]
          }
        }
        n141 = Type Cast(type="", x=w240) -> (*(type *) &x=w239:string)
        n142 = Empty String/Path?(string/path=w239) -> (empty?=w255:bool)
        n143 = Not(x=w255) -> (.not. x?=w254:bool)
      }
    }
    n144 = Cluster To Array(cluster=w97) -> (array=w100:bool[])
    n145 = Or Array Elements(Boolean array=w100) -> (logical OR=w99:bool)
    n146 = Not(x=w99) -> (.not. x?=w98:bool)
    n147 = Build Array(w98, w108, w107, w106) -> (w104:bool[])
    n148 = And Array Elements(Boolean array=w104) -> (logical AND=w105:bool)
    n149 = Not(x=w105) -> (.not. x?=w103:bool)
    n150 = call "bool to disabled state (sub-vi).vi"("error?"=w103) -> ("disabled"=w112:T24)
    n151 = property on="start button" class="Bool"(error in=w111, "DisabledEnum"=w112) -> (error out=w110:errorcluster)  [unwired: 1 in, 1 out]
    n152 = call <vilib>:"Simple Error Handler.vi"("type of dialog (OK msg:1)"=w118, "error in (no error)"=w110) -> ()  [unwired: 3 in, 5 out]
  }
  n153 = global read "global variables.vi" "sensirion subdir"() -> (w16:string)
  n154 = call <extravilib>:"Write.vi"("element"=cluster{i32, bool} {0, FALSE}) -> ("channel"=w6:T29)  [unwired: 1 out]
  n155 = call "handle input dir with subdir (subVI).vi"("subdir name (none)"=w16, "starting directory (none)"=w3) -> ("dirctory path"=w15:path)  [unwired: 8 in, 1 out]
  n156 = while {
    tunnel: w15 -> [w280]
    tunnel: w6 -> [w271]
    tunnel: w1 -> [w270]
    i -> [w279]
    stop <- w276 stop-if-true
    # "Flow Sensor Reading, Display, and Interaction"
    n157 = call <extravilib>:"Read.vi"("channel"=w270) -> ("element"=w267:bool)  [unwired: 1 in, 1 out]
    n158 = flat-sequence {
      tunnel: w279 -> [w284]
      tunnel: w280 -> [w285]
      tunnel: [w285] -> w275
      tunnel: [w284] -> w274
      tunnel: [w283] -> w273
      tunnel: [w282] -> w272
      tunnel: [w296] -> w278
      tunnel: [w303] -> w277
      tunnel: w275 -> [w298]
      tunnel: w274 -> [w294]
      tunnel: w273 -> [w303]
      tunnel: w271 -> [w302]
      tunnel: w278 -> [w318]
      tunnel: w277 -> [w315]
      tunnel: [w322] -> w268
      frame #0 {
        n159 = while {
          tunnel: [w288] -> w283
          tunnel: [w287] -> w282
          stop <- w286 stop-if-true
          n160 = event shown="[0] \"sensor monitor stop-start\": Value Change" {
            selector: _ -> [_ _]
            dyn-events: _ -> [_ _]
            timeout: _ -> [_ _]
            tunnel: [w290 w291] -> w288
            tunnel: [_ w291] -> w287
            tunnel: [w289 w291] -> w286
            event "sensor monitor stop-start": Value Change {
              n161 = event-data() -> ("NewVal"=w289:bool)  [unwired: 1 in]
              n162 = Not(x=w289) -> (.not. x?=w290:bool)
            }
            event "quit button": Value Change {
              w291 = TRUE
              n163 = event-data() -> ()  [unwired: 1 in, 1 out]
            }
          }
        }
        n164 = property on="simulate?" class="Bool (strict)"("DisabledEnum"=T24."Enabled" ("Disabled")) -> ()  [unwired: 2 in, 2 out]
      }
      frame #1 {
        n165 = call <extravilib>:"Read.vi"("channel"=w302) -> ("element"=w301:cluster{i32, bool})  [unwired: 1 in, 1 out]
        n166 = Unbundle(w301) -> (w300:i32, w293:bool)
        n167 = case shown="True" w293 {
          tunnel: w300 -> [_ w308]
          tunnel: [w305 w307] -> w295
          tunnel: w294 -> [w304 _]
          frame False {
            n168 = Format Into String(format string="flow-sensor-log_PREVIEW-%02d.csv", w304) -> (resulting string=w305:string)  [unwired: 2 in, 1 out]
          }
          frame True {
            n169 = Format Into String(format string="flow-sensor-log_stim-run-%03d.csv", w308) -> (resulting string=w307:string)  [unwired: 2 in, 1 out]
          }
        }
        n170 = property on="simulate?" class="Bool (strict)"("DisabledEnum"=T24."Disabled and Grayed Out" ("Disabled")) -> ()  [unwired: 2 in, 2 out]
        n171 = Build Path(base path=w298, name or relative path=w295) -> (appended path=w299:path)
        "flow sense path" <- w299
        n172 = Open/Create/Replace File(file path (use dialog)=w299, operation (0:open)=T30."replace or create") -> (refnum out=w296:refnum<file>)  [unwired: 4 in, 2 out]
      }
      frame #2 {
        # "reset tag channel"
        n173 = call <extravilib>:"Write.vi"("element"=FALSE) -> ("channel"=w317:T25)  [unwired: 1 out]
        n174 = while {
          tunnel: w317 -> [w403]
          tunnel: [w402] -> w322
          tunnel: w315 -> [w399]
          stop <- w401 stop-if-true
          n175 = event shown="[0] \"sensor monitor stop-start\": Value Change" {
            selector: _ -> [_ _ _]
            dyn-events: _ -> [_ _ _]
            timeout: _ -> [_ _ _]
            tunnel: [w405 w407 _] -> w404
            tunnel: [_ w407 _] -> w402
            event "sensor monitor stop-start": Value Change {
              n176 = event-data() -> ("NewVal"=w406:bool)  [unwired: 1 in]
              n177 = Not(x=w406) -> (.not. x?=w405:bool)
            }
            event "quit button": Value Change {
              w407 = TRUE
              n178 = event-data() -> ()  [unwired: 1 in, 1 out]
            }
            event Timeout {
              n179 = event-data() -> ()  [unwired: 1 in, 1 out]
            }
          }
          n180 = call "Share Stop Signal (sub-vi).vi"("set stop (F)"=w404, "channel"=w403) -> ("stop"=w400:bool)
          n181 = Or(x=w400, y=w399) -> (x .or. y?=w401:bool)
        }
        n182 = flat-sequence {
          tunnel: w318 -> [w330]
          tunnel: w317 -> [w329]
          tunnel: "Arduino COM Port" -> [w328]
          tunnel: w315 -> [w323]
          tunnel: [w327] -> w314
          tunnel: "simulate?" -> [w326]
          tunnel: [w325] -> w312
          tunnel: [TRUE] -> w311
          frame #0 {
            n183 = call "simulate or real stream sensorion data (subVI).vi"("logfile refnum"=w330, "VISA resource name (COM3)"=w328, "stop channel"=w329, "abort? (F)"=w323, "simulate?"=w326) -> ("logfile refnum out"=w325:refnum<file>, "sensor data cluster \nstream channel"=w327:T31)  [unwired: 8 in, 1 out]
          }
        }
        n184 = Close File(refnum=w312) -> ()  [unwired: 1 in, 2 out]
        n185 = call <extravilib>:"Write.vi"("element"=w311) -> ("channel"=w310:T25)  [unwired: 1 out]
        n186 = call <vilib>:"High Resolution Relative Seconds.vi"() -> ("relative seconds"=w319:dbl)
        n187 = while {
          tunnel: w314 -> [w348]
          tunnel: w315 -> [w335]
          tunnel: w319 -> [w347]
          shift-right: [w344] -> _
          shift-left: TRUE -> [w345]
          shift-right: [w342] -> _
          shift-left: w319 -> [w343]
          tunnel: w310 -> [w334]
          stop <- w331 stop-if-true
          # "only use last element from queue and valid element from queue."
          n188 = call <extravilib>:"Read.vi"("channel"=w334) -> ("element"=w333:bool)  [unwired: 1 in, 1 out]
          n189 = call <extravilib>:"Read.vi"("channel"=w348) -> ("last element?"=w336:bool, "element"=w346:T32, "element valid?"=w338:bool, "count"=w341:i32)  [unwired: 6 in, 1 out]
          n190 = Not(x=w338) -> (.not. x?=w339:bool)
          n191 = Greater Than 0?(x=w341) -> (x > 0?=w340:bool)
          n192 = Build Array(w336, w335, w333) -> (w332:bool[])
          n193 = Or(x=w339, y=w340) -> (x .or. y?=w337:bool)
          n194 = Or Array Elements(Boolean array=w332) -> (logical OR=w331:bool)
          n195 = case shown="False" w337 {
            tunnel: w346 -> [_ w365]
            tunnel: w347 -> [_ w375]
            tunnel: w345 -> [w350 w378]
            tunnel: [w350 FALSE] -> w344
            tunnel: w343 -> [w349 w374]
            tunnel: [w349 w351] -> w342
            frame True {
            }
            frame False {
              w362 = u16 2 items=["2nd Order Central", "4th Order Central", "Forward", "Backward"] ("method")
              w385 = cluster{"x":dbl, "y":dbl} {"x"=0.0, "y"=0.0} ("Point")
              n196 = Unbundle By Name(w365) -> ("relative timestamp"=w351:dbl, "sensor data array"=w393:T21[], "error"=→"Sensor Status":errorcluster)
              n197 = Subtract(x=w351, y=w375) -> (x-y=w382:dbl)
              n198 = Subtract(x=w351, y=w374) -> (x-y=w373:dbl)
              n199 = node(w382) -> (→"sensor uptime":dbl[unit])
              n200 = Array Subset(array=w393, length=10) -> (w392:T21[])  [unwired: 1 in]
              n201 = Index Array(array=w393, index #1=10 ("index")) -> (element #1=w390:T21, element #2=w389:T21)  [unwired: 1 in]
              "sensor 11 (vacuum)" <- w389
              "sensor 10 (wash)" <- w390
              n202 = Array To Cluster(array=w392) -> (cluster=→"10 sensor data clustor":T33)
              n203 = Unbundle By Name "unbundle vacuum"(w389) -> ("flow rate"=w387:dbl[unit])
              n204 = Unbundle By Name "unbundle wash"(w390) -> ("flow rate"=w386:dbl[unit])
              n205 = node(w373) -> (w372:dbl[unit])
              n206 = Subtract(x=w386, y=w387) -> (x-y=w370:dbl[unit])
              "wash-vac delta" <- w370
              n207 = node(w387) -> (w384:dbl)
              n208 = node(w386) -> (w383:dbl)
              n209 = local read "dish vol."() -> (w368:dbl[unit])
              n210 = node(w370) -> (w371:dbl)
              n211 = Multiply(x=w370, y=w372) -> (x*y=w369:dbl[unit])
              n212 = Add(x=w369, y=w368) -> (x+y=w367:dbl[unit])
              n213 = control-ref of="wash-vac delta"() -> (w388:refnum<vi>)
              n214 = call "signed value to slide format (subVI).vi"("value"=w371, "slide refnum"=w388) -> ()  [unwired: 8 in, 2 out]
              n215 = Bundle By Name(cluster=w385, "x"=w382, "y"=w384) -> (w381:cluster{"x":dbl, "y":dbl})
              n216 = Bundle By Name(cluster=w385, "x"=w382, "y"=w383) -> (w380:cluster{"x":dbl, "y":dbl})
              n217 = case shown="True" "dish volume live?" {
                tunnel: w367 -> [_ w398]
                frame False {
                }
                frame True {
                  n218 = local write "dish volume input"(w398) -> ()
                  "dish vol." <- w398
                }
              }
              n219 = Build Array(w381, w380) -> (w379:cluster{"x":dbl, "y":dbl}[])
              n220 = call "xy chart buffer (subVI).vi"("initialize buffer? (F)"=w378, "buffer length (50)"=400, "new xy point []"=w379) -> ("xy chart data []"=w352:cluster{"x":dbl[], "y":dbl[]}[])  [unwired: 7 in]
              n221 = Index Array(array=w352) -> (element=w364:cluster{"x":dbl[], "y":dbl[]})  [unwired: 1 in]
              n222 = Unbundle By Name(w364) -> ("x"=w363:dbl[])
              n223 = call "xy data array moving average (subVI).vi"("window size (3)"="mov. mean size (3)", "xy chart data []"=w352) -> ("xy chart data smooth []"=→"wash-vac flow rate \nxy graph":cluster{"x":dbl[], "y":dbl[]}[])  [unwired: 9 in]
              n224 = call <vilib>:"Derivative x(t).vi"("method"=w362, "Final Condition"=dbl[] [0.0], "X"=w363) -> ("dX/dt"=w361:dbl[])  [unwired: 7 in, 1 out]
              n225 = Delete From Array(array=w361) -> (array with subset deleted=w356:dbl[])  [unwired: 2 in, 1 out]
              n226 = call "remove nan from array (subVI).vi"("array"=w356) -> ("nan-free array"=w355:dbl[])
              n227 = call-poly <vilib>:"Mean.vi"("X"=w355) -> ("mean"=w360:dbl)  [unwired: 1 out]
              n228 = node(w360) -> (w358:dbl[unit])
              n229 = Reciprocal(x=w358) -> (1/x=→"smp rate":dbl[unit])
            }
          }
        }
      }
    }
    n230 = Build Array(w268, w272, w267) -> (w269:bool[])
    n231 = Or Array Elements(Boolean array=w269) -> (logical OR=w276:bool)
  }
  n232 = while {
    tunnel: w1 -> [w409]
    stop <- w408 stop-if-true
    # "Dish Volume Edit Interaction"
    n233 = call <extravilib>:"Read.vi"("channel"=w409) -> ("element"=w408:bool)  [unwired: 1 in, 1 out]
    n234 = event shown="[1] \"dish volume input\": Value Change" {
      selector: _ -> [_ _]
      dyn-events: _ -> [_ _]
      timeout: _ -> [_ _]
      event "dish volume live?": Value Change {
        n235 = event-data() -> ("NewVal"=w411:bool)  [unwired: 1 in]
        n236 = Not(x=w411) -> (.not. x?=w412:bool)
        n237 = call "bool to disabled state (sub-vi).vi"("error?"=w411) -> ("disabled"=w413:T24)
        n238 = call "bool to disabled state (sub-vi).vi"("error?"=w412) -> ("disabled"=w410:T24)
        n239 = property on="dish vol." class="Slide (strict)"("DisabledEnum"=w410) -> ()  [unwired: 2 in, 2 out]
        n240 = property on="dish volume input" class="DigNum (strict)"("DisabledEnum"=w413) -> ()  [unwired: 2 in, 2 out]
      }
      event "dish volume input": Value Change {
        n241 = event-data() -> ("NewVal"=w414:dbl[unit])  [unwired: 1 in]
        n242 = local write "dish vol."(w414) -> ()
      }
    }
  }
  n243 = global read "global variables.vi" "system logs subdir"() -> (w12:string)
  n244 = call "handle input dir with subdir (subVI).vi"("subdir name (none)"=w12, "starting directory (none)"=w3) -> ("dirctory path"=w11:path)  [unwired: 8 in, 1 out]
  n245 = while {
    shift-right: [w437] -> _
    shift-left: maim_stimulation_ui_states."initialize" -> [w438]
    shift-right: [w435] -> _
    shift-left: _ -> [w434]
    tunnel: w11 -> [w433]
    shift-right: [w432] -> _
    shift-left: _ -> [w431]
    shift-right: [w430] -> _
    shift-left: _ -> [w429]
    shift-right: [w420] -> _
    shift-left: _ -> [w427]
    shift-right: [w419] -> _
    shift-left: _ -> [w426]
    shift-right: [w428] -> _
    shift-left: _ -> [w425]
    shift-right: [w424] -> _
    shift-left: _ -> [w421]
    shift-right: [w423] -> _
    shift-left: _ -> [w422]
    tunnel: w6 -> [w418]
    tunnel: w1 -> [w417]
    stop <- w416 stop-if-true
    n246 = call <extravilib>:"Read.vi"("channel"=w417) -> ("element"=w415:bool)  [unwired: 1 in, 1 out]
    n247 = case shown="\"countdown\"" w438 {
      selector: w438 -> [_ w456 _ _ _ _ _ _ _ _]
      tunnel: [maim_stimulation_ui_states."wait for event" w456 maim_stimulation_ui_states."wait for event" w474 maim_stimulation_ui_states."wait for event" w497 maim_stimulation_ui_states."perform stimulation" maim_stimulation_ui_states."end stimulation" maim_stimulation_ui_states."wait for event" maim_stimulation_ui_states."idle"] -> w437
      tunnel: [_ _ _ _ _ _ _ _ _ TRUE] -> w436
      tunnel: [nan w455 w464 w473 w487 w522 w583 w599 nan w737] -> w435
      tunnel: w434 -> [_ w455 w464 w473 w487 _ w583 w599 _ w737]
      tunnel: w433 -> [_ _ _ _ _ w526 _ _ _ _]
      tunnel: [w439 w454 w463 w472 w486 "stim. run num." w582 w600 w695 w736] -> w432
      tunnel: w431 -> [_ w454 w463 w472 w486 _ w582 w600 w696 w736]
      tunnel: [refnum<k0> refnum w453 w462 w471 w485 w523 w574 w593 refnum<k0> refnum w735] -> w430
      tunnel: w429 -> [_ w453 w462 w471 w485 _ w575 w594 w708 w735]
      tunnel: [u32[] [] ("duration []") w452 w461 w470 w484 w504 w579 w590 u32[] [] ("duration []") w734] -> w419
      tunnel: [string[] [] ("description []") w451 w460 w469 w483 w517 w578 w598 string[] [] ("description []") w733] -> w428
      tunnel: w427 -> [_ w448 w457 w466 w481 _ w571 w591 _ w730]
      tunnel: w426 -> [_ w452 w461 w470 w484 _ w579 w590 _ w734]
      tunnel: w425 -> [_ w451 w460 w469 w483 _ w578 w598 _ w733]
      tunnel: [refnum<k21> refnum ("task out") w449 w458 w467 w479 w500 w572 w597 w710 w731] -> w424
      tunnel: [refnum<k21> refnum ("DAQmx Task Name") w450 w459 w468 w480 w499 w564 w595 w709 w732] -> w423
      tunnel: w422 -> [_ w450 w459 w468 w480 _ w565 w596 w709 w732]
      tunnel: w421 -> [_ w449 w458 w467 w479 _ w573 w597 w712 w731]
      tunnel: [u32[] [] ("integer []") w448 w457 w466 w481 w508 w571 w591 u32[] [] ("integer []") w730] -> w420
      tunnel: [_ _ _ _ _ w495 _ _ w700 _] -> w418
      frame "initialize", Default {
        w439 = 1
        n248 = local write "stim. run num."(w439) -> ()
      }
      frame "idle" {
      }
      frame "update listbox" {
      }
      frame "wait for event" {
        n249 = event shown="[0] \"start button\": Value Change" {
          selector: _ -> [_]
          dyn-events: _ -> [_]
          timeout: _ -> [_]
          tunnel: [w476] -> w474
          event "start button": Value Change {
            n250 = event-data() -> ()  [unwired: 1 in, 1 out]
            n251 = Select(t=maim_stimulation_ui_states."countdown", s="start button", f=maim_stimulation_ui_states."wait for event") -> (s? t:f=w476:T4)
          }
        }
      }
      frame "update nidaq task" {
      }
      frame "countdown" {
        w488 = TRUE ("Visible")
        w491 = T24."Disabled" ("Disabled")
        w490 = T24."Disabled" ("Disabled")
        w489 = T24."Disabled and Grayed Out" ("Disabled")
        n252 = flat-sequence {
          tunnel: "stim. run num." -> [w544]
          tunnel: [w541] -> w495
          frame #0 {
            n253 = Bundle("stim. run num."=w544, TRUE) -> (w542:cluster{"stim. run num.":i32, bool})  [unwired: 1 in]
            n254 = call <extravilib>:"Write.vi"("element"=w542) -> ("channel"=w541:T29)  [unwired: 1 out]
            n255 = local read "sensor monitor stop-start"() -> (w545:bool)
            n256 = case shown="False" w545 {
              frame False {
              }
              frame True {
                n257 = property on="sensor monitor stop-start" class="Bool (strict)"("Val(Sgnl)"=FALSE ("Value (Signaling)")) -> ()  [unwired: 2 in, 2 out]
              }
            }
            n258 = Wait (ms)(milliseconds to wait=u32 50) -> ()  [unwired: 1 out]
          }
          frame #1 {
            n259 = property on="sensor monitor stop-start" class="Bool (strict)"("Val(Sgnl)"=TRUE ("Value (Signaling)")) -> ()  [unwired: 2 in, 2 out]
          }
        }
        n260 = Format Into String(format string="zoss-system-log_stim-run-%03d.csv", "stim. run num.") -> (resulting string=w525:string)  [unwired: 2 in, 1 out]
        n261 = call <vilib>:"High Resolution Relative Seconds.vi"() -> ("relative seconds"=w511:dbl)
        n262 = Add(x=w511, y="pre-trig pause, s (5)") -> (x+y=w522:dbl)
        n263 = Build Path(base path=w526, name or relative path=w525) -> (appended path=w524:path)
        "stim log path" <- w524
        n264 = Open/Create/Replace File(file path (use dialog)=w524, operation (0:open)=T30."replace or create") -> (refnum out=w529:refnum<file>)  [unwired: 4 in, 2 out]
        n265 = local read "DAQmx Device Name"() -> (w501:tag)
        n266 = call "create stim logfile line (subVI).vi"("step number"=-2 ("number"), "relative seconds"=w511) -> ("string []"=w521:string[])  [unwired: 9 in]
        n267 = global read "global variables.vi" "stim logfile format"() -> (w510:string)
        n268 = Index Array(array=string[] ["rel time (s)", "step num"] ("text")) -> (element #1=w514:string, element #2=w513:string)  [unwired: 2 in]
        n269 = Format Into String(format string=w510, w514, w513) -> (resulting string=w512:string)  [unwired: 2 in, 1 out]
        n270 = case shown="\"Dev1-USB6259\"" w501 {
          tunnel: [refnum<k21> "Dev1-6259_TriggerOut_P1_L0-3" refnum<k21> refnum ("DAQmx Task Name") refnum<k21> "Sim6259_TriggerOut_P1_L0-3"] -> w500
          tunnel: [refnum<k21> "Dev1-6259_DigOut_P0" refnum<k21> refnum ("DAQmx Task Name") refnum<k21> "Sim6259_DigOut_P0"] -> w499
          tunnel: [maim_stimulation_ui_states."trigger hardware" maim_stimulation_ui_states."end stimulation" maim_stimulation_ui_states."trigger hardware"] -> w497
          frame "Dev1-USB6259" {
          }
          frame "N/A", Default {
            n271 = One Button Dialog(message="The passed DAQmx name is not supported. Please select another device.") -> ()  [unwired: 1 in, 1 out]
          }
          frame "SimDev2-USB6259" {
          }
        }
        n272 = Build Array (concatenate)(w512, w521) -> (w520:string[])
        n273 = call "append lines to loggfile (sub-vi).vi"("string array"=w520, "file refnum"=w529) -> ("file refnum out"=w523:refnum<file>)  [unwired: 8 in, 1 out]
        n274 = local read "stim. config array"() -> (w518:T5)
        n275 = property on="stim duration" class="DigNum (strict)"("DisabledEnum"=w490) -> ()  [unwired: 2 in, 2 out]
        n276 = property on="time left (s)" class="DigNum (strict)"("DisabledEnum"=w490) -> ()  [unwired: 2 in, 2 out]
        n277 = property on="config odor-manifold button" class="Bool"("DisabledEnum"=w489) -> ()  [unwired: 2 in, 2 out]
        n278 = property on="config stim button" class="Bool"("DisabledEnum"=w489) -> ()  [unwired: 2 in, 2 out]
        n279 = property on="elapsed stim. time" class="DigNum (strict)"("DisabledEnum"=w490) -> ()  [unwired: 2 in, 2 out]
        n280 = property on="DAQmx Device Name" class="DAQmxName"("DisabledEnum"=w489) -> ()  [unwired: 2 in, 2 out]
        n281 = local write "Stimulation Step"("" ("Stimulation Step")) -> ()
        n282 = local write "time left (s)"(nan ("time left (s)")) -> ()
        n283 = while {
          tunnel: w522 -> [w558]
          stop <- w557 stop-if-true
          w556 = u32 5 ("milliseconds to wait")
          n284 = Wait (ms)(milliseconds to wait=w556) -> ()  [unwired: 1 out]
          n285 = call <vilib>:"High Resolution Relative Seconds.vi"() -> ("relative seconds"=w559:dbl)
          n286 = To Double Precision Float(number=w556) -> (double precision float=w555:dbl)
          n287 = Divide(x=w555, y=1000.0) -> (x/y=w553:dbl)
          n288 = local read "est stim. time, s"() -> (w549:dbl)
          n289 = Subtract(x=w559, y=w558) -> (x-y=w550:dbl)
          "elapsed stim. time" <- w550
          n290 = Subtract(x=0.0, y=w553) -> (x-y=w551:dbl)
          n291 = Divide(x=w550, y=w549) -> (x/y=w548:dbl)
          n292 = Greater?(x=w550, y=w551) -> (0:w557:bool)
          n293 = local write "main progress bar"(w548) -> ()
        }
        n294 = call "stim config array to bool odor matrix (subVI).vi"("stim. config []"=w518) -> ("bool stim. matrix"=w509:bool[][], "duration []"=w506:dbl[])  [unwired: 8 in, 1 out]
        n295 = property on="main progress bar" class="Slide (strict)"("Visible"=w488) -> ()  [unwired: 2 in, 2 out]
        n296 = property on="stim progress bar" class="Slide (strict)"("Visible"=w488) -> ()  [unwired: 2 in, 2 out]
        n297 = call "stim config array to description array (subVI).vi"("add index? (F)"=TRUE, "stim. config array"=w518) -> ("description []"=w517:string[])  [unwired: 9 in]
        n298 = call "bool 2d array to uint array.vi"("bool [] []"=w509) -> ("integer []"=w508:u32[])
        n299 = property on="trig off btn" class="Bool (strict)"("DisabledEnum"=w489) -> ()  [unwired: 2 in, 2 out]
        n300 = property on="trig on btn" class="Bool (strict)"("DisabledEnum"=w489) -> ()  [unwired: 2 in, 2 out]
        n301 = property on="sol. off btn." class="Bool (strict)"("DisabledEnum"=w489) -> ()  [unwired: 2 in, 2 out]
        n302 = Multiply(x=w506, y=1000.0) -> (x*y=w507:dbl[])
        n303 = local write "stim status mc listbox"(-1 ("stim status mc listbox")) -> ()
        n304 = To Unsigned Long Integer(number=w507) -> (unsigned 32bit integer=w504:u32[])
        n305 = property on="stim. run num." class="DigNum (strict)"("DisabledEnum"=T24."Disabled and Grayed Out" ("Disabled"), "Caption.Text"="Stimulation Run Index") -> ()  [unwired: 2 in, 2 out]
        n306 = property on="Solenoid Status" class="Clust (strict)"("DisabledEnum"=w491) -> ()  [unwired: 2 in, 2 out]
        n307 = property on="Stimulation Step" class="Str"("DisabledEnum"=w491) -> ()  [unwired: 2 in, 2 out]
        n308 = property on="start button" class="Bool"("DisabledEnum"=w489) -> ()  [unwired: 2 in, 2 out]
        n309 = property on="Trigger Selection" class="Clust (strict)"("DisabledEnum"=w489) -> ()  [unwired: 2 in, 2 out]
      }
      frame "trigger hardware" {
        w567 = u32 0 ("number")
        n310 = Number To Boolean Array(number=w567) -> (Boolean array=w570:bool[])
        n311 = call-poly <vilib>:"DAQmx Write.vi"("task/channels in"=w565, "auto start"=TRUE, "data"=w567) -> ("task out"=w564:refnum<k21>)  [unwired: 10 in, 2 out]
        n312 = Array Subset(array=w570, length=10) -> (w569:bool[])  [unwired: 1 in]
        n313 = Array To Cluster(array=w569) -> (cluster=w568:T28)
        n314 = local write "Solenoid Status"(w568) -> ()
        n315 = Cluster To Array(cluster="Trigger Selection") -> (array=w561:bool[])
        n316 = flat-sequence {
          tunnel: w561 -> [w586]
          tunnel: [w588] -> w576
          tunnel: w573 -> [w587]
          tunnel: [w585] -> w572
          frame #0 {
            n317 = call-poly <vilib>:"DAQmx Write.vi"("task/channels in"=w587, "auto start"=TRUE, "data"=w586) -> ("task out"=w585:refnum<k21>)  [unwired: 10 in, 2 out]
            n318 = call <vilib>:"High Resolution Relative Seconds.vi"() -> ("relative seconds"=w588:dbl)
          }
        }
        n319 = Array To Cluster(array=w561) -> (cluster=→"Triggers":T35)
        n320 = call "create stim logfile line (subVI).vi"("step number"=-1, "relative seconds"=w576) -> ("string []"=w577:string[])  [unwired: 9 in]
        n321 = call "append lines to loggfile (sub-vi).vi"("string array"=w577, "file refnum"=w575) -> ("file refnum out"=w574:refnum<file>)  [unwired: 8 in, 1 out]
      }
      frame "perform stimulation" {
        n322 = Array Size(array=w591) -> (size(s)=w589:i32)
        n323 = while {
          tunnel: w591 -> [w613] mode=indexing
          tunnel: w590 -> [w609] mode=indexing
          tunnel: w598 -> [w610] mode=indexing
          shift-right: [w614] -> w595
          shift-left: w596 -> [w615]
          shift-right: [w611] -> w593
          shift-left: w594 -> [w612]
          tunnel: [w607] -> w592
          tunnel: w589 -> [w606]
          i -> [w605]
          stop <- w603 stop-if-true
          n324 = Greater?(x=w606, y=w605) -> (0:w604:bool)
          n325 = case shown="True" w604 {
            tunnel: w615 -> [w622 w654]
            tunnel: [w621 w653] -> w614
            tunnel: w613 -> [_ w652]
            tunnel: w612 -> [w620 w646]
            tunnel: [w619 w645] -> w611
            tunnel: w610 -> [_ w644]
            tunnel: w609 -> [_ _]
            tunnel: [T34 {"valid?"=FALSE, "rel. time, s"=0.0, "index"=0} ("stim timestamp cluster") w640] -> w608
            tunnel: w605 -> [_ w639]
            tunnel: [TRUE _] -> w603
            frame False {
              w625 = u32 0 ("number")
              n326 = Number To Boolean Array(number=w625) -> (Boolean array=w631:bool[])
              n327 = flat-sequence {
                tunnel: w622 -> [w638]
                tunnel: [w637] -> w621
                tunnel: w625 -> [w636]
                tunnel: [w635] -> w628
                frame #0 {
                  n328 = call <vilib>:"High Resolution Relative Seconds.vi"() -> ("relative seconds"=w635:dbl)
                  n329 = call-poly <vilib>:"DAQmx Write.vi"("task/channels in"=w638, "auto start"=TRUE, "data"=w636) -> ("task out"=w637:refnum<k21>)  [unwired: 10 in, 2 out]
                }
              }
              n330 = local write "Stimulation Step"("" ("Stimulation Step")) -> ()
              n331 = local write "stim duration"(nan ("stim duration")) -> ()
              n332 = local write "stim status mc listbox"(-1 ("stim status mc listbox")) -> ()
              n333 = Array Subset(array=w631, length=10) -> (w630:bool[])  [unwired: 1 in]
              n334 = Array To Cluster(array=w630) -> (cluster=w627:T28)
              n335 = local write "Solenoid Status"(w627) -> ()
              n336 = call "create stim logfile line (subVI).vi"("step number"=-3, "relative seconds"=w628) -> ("string []"=w629:string[])  [unwired: 9 in]
              n337 = call "append lines to loggfile (sub-vi).vi"("string array"=w629, "file refnum"=w620) -> ("file refnum out"=w619:refnum<file>)  [unwired: 8 in, 1 out]
            }
            frame True {
              n338 = Number To Boolean Array(number=w652) -> (Boolean array=w651:bool[])
              n339 = flat-sequence {
                tunnel: w654 -> [w659]
                tunnel: [w658] -> w653
                tunnel: w652 -> [w657]
                tunnel: [w656] -> w641
                frame #0 {
                  n340 = call <vilib>:"High Resolution Relative Seconds.vi"() -> ("relative seconds"=w656:dbl)
                  n341 = call-poly <vilib>:"DAQmx Write.vi"("task/channels in"=w659, "auto start"=TRUE, "data"=w657) -> ("task out"=w658:refnum<k21>)  [unwired: 10 in, 2 out]
                }
              }
              n342 = Array Subset(array=w651, length=10) -> (w649:bool[])  [unwired: 1 in]
              n343 = Array To Cluster(array=w649) -> (cluster=→"Solenoid Status":T28)
              n344 = call "create stim logfile line (subVI).vi"("step number"=w639, "relative seconds"=w641) -> ("string []"=w647:string[])  [unwired: 9 in]
              n345 = Bundle By Name(cluster=T34 {"valid?"=FALSE, "rel. time, s"=0.0, "index"=0} ("stim timestamp cluster"), "valid?"=TRUE, "rel. time, s"=w641, "index"=w639) -> (w640:T34)
              n346 = call "append lines to loggfile (sub-vi).vi"("string array"=w647, "file refnum"=w646) -> ("file refnum out"=w645:refnum<file>)  [unwired: 8 in, 1 out]
              "Stimulation Step" <- w644
              "stim status mc listbox" <- w639
            }
          }
          n347 = case shown="True" w604 {
            tunnel: w609 -> [_ w616]
            frame False {
            }
            frame True {
              n348 = Wait (ms)(milliseconds to wait=w616) -> ()  [unwired: 1 out]
            }
          }
          n349 = call <extravilib>:"Write With Abort.vi"("abort"=w603, "element"=w608) -> ("channel"=w607:T36)  [unwired: 7 in, 2 out]
        }
        n350 = while {
          tunnel: w599 -> [w673]
          tunnel: w592 -> [w671]
          tunnel: w590 -> [w668]
          stop <- w664 stop-if-true
          n351 = call <extravilib>:"Read With Abort.vi"("abort"=FALSE ("abort (F)"), "channel"=w671) -> ("element"=w670:T34, "aborted?"=w664:bool)  [unwired: 7 in, 1 out]
          n352 = Unbundle By Name(w670) -> ("index"=w669:i32, "rel. time, s"=w667:dbl, "valid?"=w665:bool)
          n353 = call <vilib>:"High Resolution Relative Seconds.vi"() -> ("relative seconds"=w666:dbl)
          n354 = Wait (ms)(milliseconds to wait=u32 5) -> ()  [unwired: 1 out]
          n355 = Subtract(x=w666, y=w673) -> (x-y=w661:dbl)
          n356 = case shown="True" w665 {
            tunnel: w669 -> [_ w687]
            tunnel: w668 -> [_ w686]
            tunnel: w667 -> [_ w683]
            tunnel: w666 -> [_ w682]
            frame False {
              w675 = T24."Disabled and Grayed Out" ("Disabled")
              w674 = nan ("time left (s)")
              n357 = local write "time left (s)"(w674) -> ()
              n358 = local write "stim duration"(w674) -> ()
              n359 = property on="time left (s)" class="DigNum (strict)"("DisabledEnum"=w675) -> ()  [unwired: 2 in, 2 out]
              n360 = property on="stim duration" class="DigNum (strict)"("DisabledEnum"=w675) -> ()  [unwired: 2 in, 2 out]
            }
            frame True {
              w679 = T24."Disabled" ("Disabled")
              n361 = Index Array(array=w686, index=w687) -> (element=w684:u32)
              n362 = To Double Precision Float(number=w684) -> (double precision float=w681:dbl)
              n363 = Subtract(x=w683, y=w682) -> (x-y=w685:dbl)
              n364 = Divide(x=w681, y=1000.0) -> (x/y=w677:dbl)
              "stim duration" <- w677
              n365 = property on="time left (s)" class="DigNum (strict)"("DisabledEnum"=w679) -> ()  [unwired: 2 in, 2 out]
              n366 = property on="stim duration" class="DigNum (strict)"("DisabledEnum"=w679) -> ()  [unwired: 2 in, 2 out]
              n367 = Add(x=w685, y=w677) -> (x+y=w678:dbl)
              "time left (s)" <- w678
              n368 = Divide(x=w678, y=w677) -> (x/y=→"stim progress bar":dbl)
            }
          }
          n369 = local read "est stim. time, s"() -> (w660:dbl)
          n370 = local write "elapsed stim. time"(w661) -> ()
          n371 = Divide(x=w661, y=w660) -> (x/y=→"main progress bar":dbl)
        }
        "stimulation" <- TRUE ("stimulation")
      }
      frame "end stimulation" {
        w688 = FALSE ("Visible")
        w689 = T24."Enabled" ("Disabled")
        w690 = 0.0 ("main progress bar")
        w692 = T24."Enabled" ("Disabled")
        w722 = T24."Enabled" ("Disabled")
        n372 = Increment(x=w696) -> (x+1=w695:i32)
        n373 = Close File(refnum=w708) -> ()  [unwired: 1 in, 2 out]
        n374 = local write "stim. run num."(w695) -> ()
        n375 = local write "stimulation"(FALSE ("stimulation")) -> ()
        n376 = local write "stim duration"(nan ("stim duration")) -> ()
        n377 = local write "time left (s)"(nan ("time left (s)")) -> ()
        n378 = property on="time left (s)" class="DigNum (strict)"("DisabledEnum"=T24."Disabled and Grayed Out" ("Disabled")) -> ()  [unwired: 2 in, 2 out]
        n379 = property on="config odor-manifold button" class="Bool"("DisabledEnum"=w722) -> ()  [unwired: 2 in, 2 out]
        n380 = property on="config stim button" class="Bool"("DisabledEnum"=w722) -> ()  [unwired: 2 in, 2 out]
        n381 = local write "stim status mc listbox"(-1 ("stim status mc listbox")) -> ()
        n382 = property on="DAQmx Device Name" class="DAQmxName"("DisabledEnum"=T24."Enabled" ("Disabled")) -> ()  [unwired: 2 in, 2 out]
        n383 = property on="stim duration" class="DigNum (strict)"("DisabledEnum"=T24."Disabled and Grayed Out" ("Disabled")) -> ()  [unwired: 2 in, 2 out]
        n384 = property on="Solenoid Status" class="Clust (strict)"("DisabledEnum"=T24."Disabled and Grayed Out" ("Disabled")) -> ()  [unwired: 2 in, 2 out]
        n385 = property on="Stimulation Step" class="Str"("DisabledEnum"=T24."Disabled and Grayed Out" ("Disabled")) -> ()  [unwired: 2 in, 2 out]
        n386 = property on="main progress bar" class="Slide (strict)"("Visible"=w688, "Value"=w690) -> ()  [unwired: 2 in, 2 out]
        n387 = property on="stim progress bar" class="Slide (strict)"("Visible"=w688, "Value"=w690) -> ()  [unwired: 2 in, 2 out]
        n388 = flat-sequence {
          frame #0 {
            n389 = call <vilib>:"Set Busy.vi"() -> ()  [unwired: 10 in, 2 out]
            n390 = Multiply(x=1000.0, y="post-stim pause, s (3)") -> (x*y=w725:dbl)
            n391 = To Unsigned Long Integer(number=w725) -> (unsigned 32bit integer=w724:u32)
            n392 = Wait (ms)(milliseconds to wait=w724) -> ()  [unwired: 1 out]
          }
          frame #1 {
            n393 = property on="sensor monitor stop-start" class="Bool (strict)"("Val(Sgnl)"=FALSE ("Value (Signaling)")) -> ()  [unwired: 2 in, 2 out]
            n394 = property on="elapsed stim. time" class="DigNum (strict)"("DisabledEnum"=T24."Disabled and Grayed Out" ("Disabled")) -> ()  [unwired: 2 in, 2 out]
            n395 = call <vilib>:"Unset Busy.vi"() -> ()  [unwired: 11 in, 1 out]
          }
        }
        n396 = property on="trig off btn" class="Bool (strict)"("DisabledEnum"=w692) -> ()  [unwired: 2 in, 2 out]
        n397 = property on="trig on btn" class="Bool (strict)"("DisabledEnum"=w692) -> ()  [unwired: 2 in, 2 out]
        n398 = property on="sol. off btn." class="Bool (strict)"("DisabledEnum"=w692) -> ()  [unwired: 2 in, 2 out]
        n399 = property on="start button" class="Bool"("DisabledEnum"=w689) -> ()  [unwired: 2 in, 2 out]
        n400 = property on="Trigger Selection" class="Clust (strict)"("DisabledEnum"=w689) -> ()  [unwired: 2 in, 2 out]
        n401 = property on="stim. run num." class="DigNum (strict)"("DisabledEnum"=T24."Enabled" ("Disabled"), "Caption.Text"="Next Stimulation Run Index") -> ()  [unwired: 2 in, 2 out]
        n402 = Initialize Array(FALSE, 4 ("dimension size")) -> (w711:bool[])
        n403 = Array To Cluster(array=w711) -> (cluster=w718:T27)
        n404 = call-poly <vilib>:"DAQmx Write.vi"("task/channels in"=w712, "data"=w711) -> ("task out"=w710:refnum<k21>)  [unwired: 11 in, 2 out]
        n405 = local write "Triggers"(w718) -> ()
        n406 = Bundle(0, FALSE) -> (w699:cluster{i32, bool})  [unwired: 1 in]
        n407 = call <extravilib>:"Write.vi"("element"=w699) -> ("channel"=w700:T29)  [unwired: 1 out]
      }
      frame "exit" {
      }
    }
    n408 = Or(x=w436, y=w415) -> (x .or. y?=w416:bool)
    "stim loop state" <- w438
  }
  n409 = global read "global variables.vi" "system logs subdir"() -> (w4:string)
  n410 = call "handle input dir with subdir (subVI).vi"("subdir name (none)"=w4, "starting directory (none)"=w3) -> ("dirctory path"=w2:path)  [unwired: 8 in, 1 out]
  n411 = while {
    tunnel: w6 -> [w744]
    tunnel: w1 -> [w750]
    shift-right: [w749] -> _
    shift-left: w2 -> [w751]
    shift-right: [w748] -> _
    shift-left: cam_2p_status_logging_states."initialize" ("Enum") -> [w752]
    shift-right: [w743] -> _
    shift-left: _ -> [w742]
    shift-right: [w741] -> _
    shift-left: _ -> [w740]
    stop <- w747 stop-if-true
    # "Sync Status Logging Loop"
    n412 = call <extravilib>:"Read.vi"("channel"=w750) -> ("element"=w746:bool)  [unwired: 1 in, 1 out]
    n413 = case shown="\"prepare for log\"" w752 {
      tunnel: w751 -> [w756 w759 w760 w775 _ _ _]
      tunnel: [w756 w759 w760 w775 _ _ _] -> w749
      tunnel: [cam_2p_status_logging_states."idle" ("Enum") cam_2p_status_logging_states."wait for stim begin" ("Enum") w761 cam_2p_status_logging_states."log" ("f") _ _ _] -> w748
      tunnel: [FALSE ("x") _ _ _ _ _ _] -> w745
      tunnel: w744 -> [_ _ w767 _ _ _ _]
      tunnel: [-1 _ w765 w776 _ -1 _] -> w743
      tunnel: w742 -> [_ _ _ w776 _ _ _]
      tunnel: [_ _ _ w777 _ _ _] -> w741
      tunnel: w740 -> [_ _ _ _ _ _ _]
      frame "initialize", Default {
      }
      frame "idle" {
        n414 = Wait (ms)(milliseconds to wait=u32 10) -> ()  [unwired: 1 out]
      }
      frame "wait for stim begin" {
        n415 = call <extravilib>:"Read.vi"("channel"=w767) -> ("element"=w766:cluster{i32, bool})  [unwired: 1 in, 1 out]
        n416 = Unbundle(w766) -> (w765:i32, w764:bool)
        n417 = Select(t=cam_2p_status_logging_states."prepare for log" ("Enum"), s=w764, f=cam_2p_status_logging_states."idle") -> (s? t:f=w761:T22)
      }
      frame "prepare for log" {
        n418 = global read "global variables.vi" "cam and 2p status logfile format"() -> (w790:string)
        n419 = Format Into String(format string="zoss-cam-2p-status-log_stim-run-%03d.csv", w776) -> (resulting string=w784:string)  [unwired: 2 in, 1 out]
        n420 = Index Array(array=string[] ["rel time (s)", "2p status", "cam status"] ("text")) -> (element #1=w787:string, element #2=w786:string, element #3=w785:string)  [unwired: 3 in]
        n421 = Build Path(base path=w775, name or relative path=w784) -> (appended path=w783:path)
        n422 = Format Into String(format string=w790, w787, w786, w785) -> (resulting string=w780:string)  [unwired: 2 in, 1 out]
        n423 = Open/Create/Replace File(file path (use dialog)=w783, operation (0:open)=T30."replace or create") -> (refnum out=w779:refnum<file>)  [unwired: 4 in, 2 out]
        n424 = Build Array(w780) -> (w778:string[])
        n425 = call "append lines to loggfile (sub-vi).vi"("string array"=w778, "file refnum"=w779) -> ("file refnum out"=w777:refnum<file>)  [unwired: 8 in, 1 out]
        n426 = local read "DAQmx Device Name 2"() -> (w774:tag)
        n427 = local read "DAQmx Device Name 3"() -> (w772:tag)
        n428 = case shown="\"Dev1-USB6259\"" w774 {
          tunnel: [refnum<k21> "Dev1-6259_TriggerOut_P1_L0-3" refnum<k21> refnum ("DAQmx Task Name") refnum<k21> "Sim6259_TriggerOut_P1_L0-3"] -> w773
          tunnel: [refnum<k21> "Dev1-6259_DigOut_P0" refnum<k21> refnum ("DAQmx Task Name") refnum<k21> "Sim6259_DigOut_P0"] -> _
          tunnel: [maim_stimulation_ui_states."trigger hardware" maim_stimulation_ui_states."end stimulation" maim_stimulation_ui_states."trigger hardware"] -> _
          frame "Dev1-USB6259" {
          }
          frame "N/A", Default {
            n429 = One Button Dialog(message="The passed DAQmx name is not supported. Please select another device.") -> ()  [unwired: 1 in, 1 out]
          }
          frame "SimDev2-USB6259" {
          }
        }
        n430 = local read "DAQmx Device Name 4"() -> (w770:tag)
        n431 = local read "DAQmx Device Name 5"() -> (w768:tag)
        n432 = case shown="\"Dev1-USB6259\"" w772 {
          tunnel: [refnum<k21> "Dev1-6259_TriggerOut_P1_L0-3" refnum<k21> refnum ("DAQmx Task Name") refnum<k21> "Sim6259_TriggerOut_P1_L0-3"] -> w771
          tunnel: [refnum<k21> "Dev1-6259_DigOut_P0" refnum<k21> refnum ("DAQmx Task Name") refnum<k21> "Sim6259_DigOut_P0"] -> _
          tunnel: [maim_stimulation_ui_states."trigger hardware" maim_stimulation_ui_states."end stimulation" maim_stimulation_ui_states."trigger hardware"] -> _
          frame "Dev1-USB6259" {
          }
          frame "N/A", Default {
            n433 = One Button Dialog(message="The passed DAQmx name is not supported. Please select another device.") -> ()  [unwired: 1 in, 1 out]
          }
          frame "SimDev2-USB6259" {
          }
        }
        n434 = case shown="\"Dev1-USB6259\"" w770 {
          tunnel: [refnum<k21> "Dev1-6259_TriggerOut_P1_L0-3" refnum<k21> refnum ("DAQmx Task Name") refnum<k21> "Sim6259_TriggerOut_P1_L0-3"] -> w769
          tunnel: [refnum<k21> "Dev1-6259_DigOut_P0" refnum<k21> refnum ("DAQmx Task Name") refnum<k21> "Sim6259_DigOut_P0"] -> _
          tunnel: [maim_stimulation_ui_states."trigger hardware" maim_stimulation_ui_states."end stimulation" maim_stimulation_ui_states."trigger hardware"] -> _
          frame "Dev1-USB6259" {
          }
          frame "N/A", Default {
            n435 = One Button Dialog(message="The passed DAQmx name is not supported. Please select another device.") -> ()  [unwired: 1 in, 1 out]
          }
          frame "SimDev2-USB6259" {
          }
        }
        n436 = case shown="\"Dev1-USB6259\"" w768 {
          tunnel: [refnum<k21> "Dev1-6259_TriggerOut_P1_L0-3" refnum<k21> refnum ("DAQmx Task Name") refnum<k21> "Sim6259_TriggerOut_P1_L0-3"] -> _
          tunnel: [refnum<k21> "Dev1-6259_DigOut_P0" refnum<k21> refnum ("DAQmx Task Name") refnum<k21> "Sim6259_DigOut_P0"] -> _
          tunnel: [maim_stimulation_ui_states."trigger hardware" maim_stimulation_ui_states."end stimulation" maim_stimulation_ui_states."trigger hardware"] -> _
          frame "Dev1-USB6259" {
          }
          frame "N/A", Default {
            n437 = One Button Dialog(message="The passed DAQmx name is not supported. Please select another device.") -> ()  [unwired: 1 in, 1 out]
          }
          frame "SimDev2-USB6259" {
          }
        }
        n438 = local read "DAQmx Device Name 6"() -> ()  [unwired: 1 out]
        n439 = local read "DAQmx Device Name 7"() -> ()  [unwired: 1 out]
      }
      frame "log" {
      }
      frame "end log" {
      }
      frame "exit" {
      }
    }
    n440 = Or(x=w745, y=w746) -> (x .or. y?=w747:bool)
  }
